vi "Get_Vertical_Scale.vi"(7 "error in (no error)":errorcluster, 9 "Active_Channels":u16[](array[numeric]), 10 "VISA resource name":refnum<visa-resource-name>="Master_Oscilloscope") -> (0 "error out":errorcluster, 2 "Vertical_Parameters":string[](array[string]), 3 "VISA resource name out":refnum<visa-resource-name>)   [LabVIEW 2020]
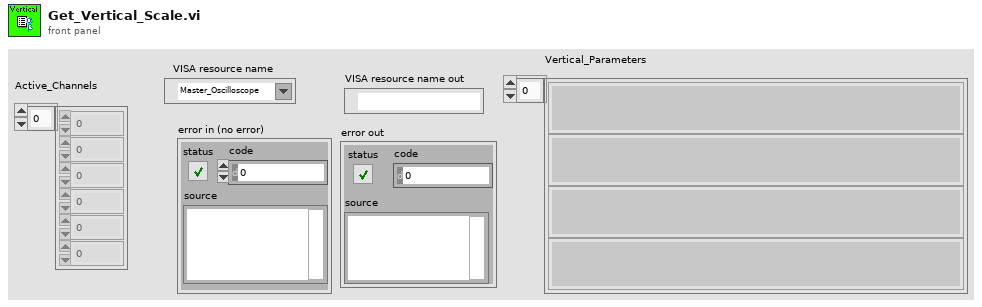
[diagram p1: front panel]
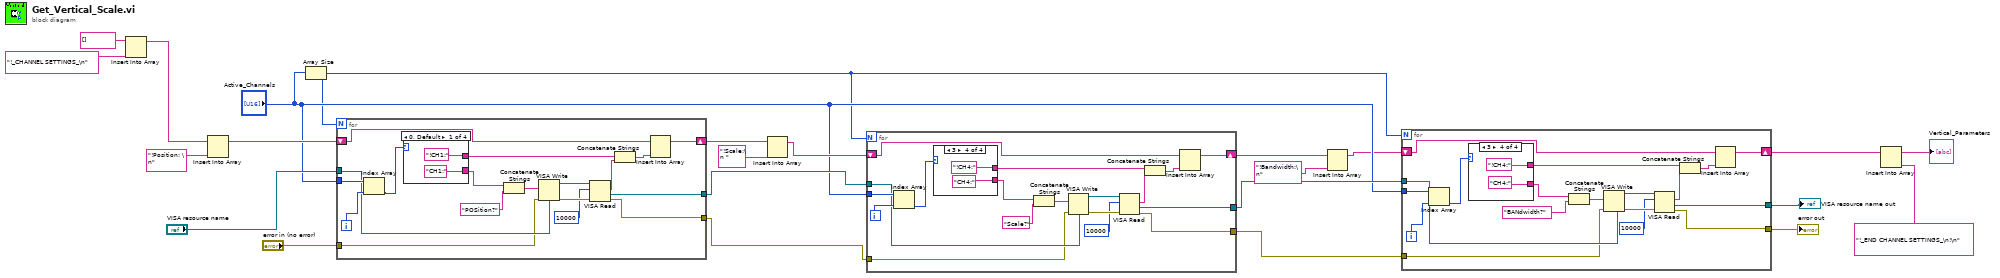
[diagram p0: block diagram]
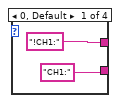
[diagram p2: hidden frame]
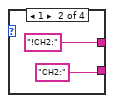
[diagram p3: hidden frame]
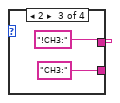
[diagram p4: hidden frame]
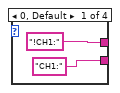
[diagram p5: hidden frame]
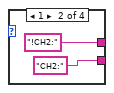
[diagram p6: hidden frame]
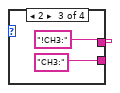
[diagram p7: hidden frame]
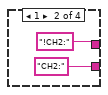
[diagram p8: hidden frame]
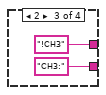
[diagram p9: hidden frame]
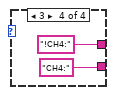
[diagram p10: hidden frame]
diagram:
  n1 = Insert Into Array(array=string[] [], new element="!_CHANNEL SETTINGS_\n") -> (w21:string[])  [unwired: 1 in]
  n2 = Insert Into Array(array=w21, new element="!Position: \n") -> (w19:string[])  [unwired: 1 in]
  n3 = Array Size(array="Active_Channels") -> (size(s)=w9:i32)
  n4 = for {
    N: w9 -> [_]
    tunnel: "Active_Channels" -> [w35]
    tunnel: "VISA resource name" -> [w33]
    tunnel: [w32] -> w17
    tunnel: [w31] -> w18
    tunnel: "error in (no error)" -> [w30]
    shift-right: [w27] -> w16
    shift-left: w19 -> [w28]
    i -> [w36]
    n5 = Index Array(array=w35, index=w36) -> (element=w34:u16)
    n6 = case shown="0, Default" w34 {
      tunnel: ["CH1:" "CH2:" "CH3:" "CH4:"] -> w26
      tunnel: ["!CH1:" "!CH2:" "!CH3" "!CH4:"] -> w25
      frame 0, Default {
      }
      frame 1 {
      }
      frame 2 {
      }
      frame 3 {
      }
    }
    n7 = Concatenate Strings(w26, "POSition?" ("write buffer")) -> (w41:string)
    n8 = VISA Write(VISA resource name=w33, write buffer=w41, error in (no error)=w30) -> (VISA resource name out=w40:refnum<visa-resource-name>, error out=w39:errorcluster)  [unwired: 1 out]
    n9 = VISA Read(VISA resource name=w40, byte count=u32 10000, error in (no error)=w39) -> (VISA resource name out=w32:refnum<visa-resource-name>, read buffer=w37:string, error out=w31:errorcluster)  [unwired: 1 out]
    n10 = Concatenate Strings(w25, w37) -> (w29:string)
    n11 = Insert Into Array(array=w28, new element=w29) -> (w27:string[])  [unwired: 1 in]
  }
  n12 = Insert Into Array(array=w16, new element="!Scale:\n ") -> (w15:string[])  [unwired: 1 in]
  n13 = for {
    N: w9 -> [_]
    tunnel: "Active_Channels" -> [w61]
    tunnel: w17 -> [w59]
    tunnel: [w58] -> w11
    tunnel: [w57] -> w8
    tunnel: w18 -> [w56]
    shift-right: [w52] -> w7
    shift-left: w15 -> [w53]
    i -> [w62]
    n14 = Index Array(array=w61, index=w62) -> (element=w60:u16)
    n15 = case shown="3" w60 {
      tunnel: ["!CH1:" "!CH2:" "!CH3:" "!CH4:"] -> w55
      tunnel: ["CH1:" "CH2:" "CH3:" "CH4:"] -> w51
      frame 0, Default {
      }
      frame 1 {
      }
      frame 2 {
      }
      frame 3 {
      }
    }
    n16 = Concatenate Strings(w51, "Scale?" ("write buffer")) -> (w67:string)
    n17 = VISA Write(VISA resource name=w59, write buffer=w67, error in (no error)=w56) -> (VISA resource name out=w66:refnum<visa-resource-name>, error out=w65:errorcluster)  [unwired: 1 out]
    n18 = VISA Read(VISA resource name=w66, byte count=u32 10000, error in (no error)=w65) -> (VISA resource name out=w58:refnum<visa-resource-name>, read buffer=w63:string, error out=w57:errorcluster)  [unwired: 1 out]
    n19 = Concatenate Strings(w55, w63) -> (w54:string)
    n20 = Insert Into Array(array=w53, new element=w54) -> (w52:string[])  [unwired: 1 in]
  }
  n21 = Insert Into Array(array=w7, new element="!Bandwidth:\n") -> (w5:string[])  [unwired: 1 in]
  n22 = for {
    N: w9 -> [_]
    tunnel: "Active_Channels" -> [w88]
    tunnel: w11 -> [w86]
    tunnel: [w85] -> w13
    tunnel: [w84] -> w12
    tunnel: w8 -> [w83]
    shift-right: [w79] -> w4
    shift-left: w5 -> [w80]
    i -> [w89]
    n23 = Index Array(array=w88, index=w89) -> (element=w87:u16)
    n24 = case shown="3" w87 {
      tunnel: ["!CH1:" "!CH2:" "!CH3:" "!CH4:"] -> w82
      tunnel: ["CH1:" "CH2:" "CH3:" "CH4:"] -> w77
      frame 0, Default {
      }
      frame 1 {
      }
      frame 2 {
      }
      frame 3 {
      }
    }
    n25 = Concatenate Strings(w77, "BANdwidth?" ("write buffer")) -> (w94:string)
    n26 = VISA Write(VISA resource name=w86, write buffer=w94, error in (no error)=w83) -> (VISA resource name out=w93:refnum<visa-resource-name>, error out=w92:errorcluster)  [unwired: 1 out]
    n27 = VISA Read(VISA resource name=w93, byte count=u32 10000, error in (no error)=w92) -> (VISA resource name out=w85:refnum<visa-resource-name>, read buffer=w90:string, error out=w84:errorcluster)  [unwired: 1 out]
    n28 = Concatenate Strings(w82, w90) -> (w81:string)
    n29 = Insert Into Array(array=w80, new element=w81) -> (w79:string[])  [unwired: 1 in]
  }
  "error out" <- w12
  "VISA resource name out" <- w13
  n30 = Insert Into Array(array=w4, new element="!_END CHANNEL SETTINGS_\n!\n") -> (→"Vertical_Parameters":string[])  [unwired: 1 in]
